vi "COM_Sort_Modes.vi"(7 "Mode":T2, 8 "Error In":errorcluster, 10 "Modes In":T1[](array[typedef]), 11 "Mode Records In":refnum<class "Mode.lvclass">[](array[class])) -> (0 "Error Out":errorcluster, 2 "Modes Out":T1[](array[typedef]), 3 "Mode Records Out":refnum<class "Mode.lvclass">[](array[class]))   [LabVIEW 2017, in "AppPlugins.lvlib" / "EraPlugin.lvclass"]
uses:
  EraPlugin.lvclass
  Mode/Mode.lvclass
  Mode/Mode Content.ctl
  Mode/Mode_Type.ctl
panel:
  in  "Retirement (s)":dbl=30.0 format="%#_13g"
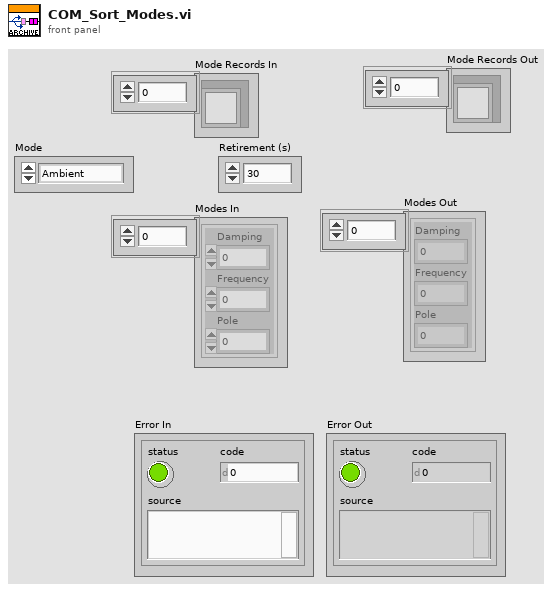
[diagram p1: front panel]
types:
  T1 = typedef "Mode.lvclass/Mode Content.ctl" = cluster{"Damping":dbl, "Frequency":dbl, "Pole":cdb}
  T2 = typedef "Mode.lvclass/Mode_Type.ctl" = enum16{"Ambient", "ERA"}
  T3 = cluster{"avg_f":dbl, "sigma_f":dbl, "avg_d":dbl, "sigma_d":dbl}
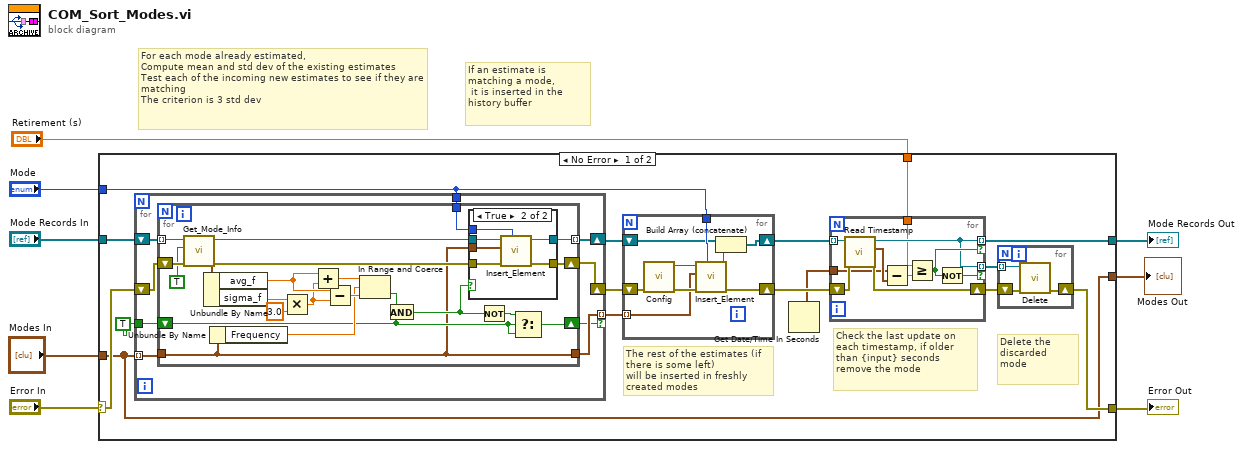
[diagram p0: block diagram]
diagram:
  # "If an estimate is matching a mode,\n it is inserted in the history buffer"
  # "For each mode already estimated,\nCompute mean and std dev of the existing estimates\nTest each of the incoming new estimates to see if they are matching\nThe criterion is 3 std dev"
  n1 = case shown="No Error" "Error In" {
    selector: "Error In" -> [w19 w88]
    tunnel: "Mode Records In" -> [w24 w87]
    tunnel: [w16 w87] -> w7
    tunnel: "Mode" -> [w21 _]
    tunnel: [w12 w88] -> w5
    tunnel: [w9 w86] -> w3
    tunnel: "Retirement (s)" -> [w11 _]
    tunnel: "Modes In" -> [w9 w86]
    frame No Error {
      # "Delete the discarded mode"
      # "Check the last update on each timestamp, if older than {input} seconds remove the mode"
      # "The rest of the estimates (if there is some left) \nwill be inserted in freshly created modes"
      n2 = for {
        shift-right: [w54] -> w22
        shift-left: w19 -> [w51]
        tunnel: w21 -> [w55]
        tunnel: TRUE ("x .and. y?") -> [w53]
        shift-right: [w50] -> w23
        shift-left: w24 -> [w52]
        tunnel: w9 -> [w49] mode=indexing
        tunnel: [w48] -> w10 mode=indexing if=w47
        n3 = for {
          tunnel: w55 -> [w74]
          shift-right: [w73] -> w54
          shift-left: w51 -> [w68]
          shift-right: [w72] -> w47
          shift-left: w53 -> [w62]
          tunnel: w52 -> [w70] mode=indexing
          tunnel: [w65] -> w50 mode=indexing
          tunnel: w49 -> [w56]
          tunnel: [w56] -> w48
          n4 = call "Get_Mode_Info.vi"("Error In"=w68, "Coerce?"=TRUE, "Input"=w70) -> ("Error Out"=w67:errorcluster, "Modes_info"=w66:T3, "Output"=w69:refnum<class "Mode.lvclass">)  [unwired: 5 in, 1 out]
          n5 = Unbundle By Name(w66) -> ("avg_f"=w77:dbl, "sigma_f"=w59:dbl)
          n6 = Unbundle By Name(w56) -> ("Frequency"=w64:dbl)
          n7 = Multiply(x=w59, y=3.0) -> (x*y=w58:dbl)
          n8 = Add(x=w77, y=w58) -> (x+y=w75:dbl)
          n9 = Subtract(x=w77, y=w58) -> (x-y=w76:dbl)
          n10 = In Range and Coerce(upper limit=w75, x=w64, lower limit=w76) -> (In Range?=w63:bool)  [unwired: 1 out]
          n11 = And(x=w63, y=w62) -> (x .and. y?=w61:bool)
          n12 = case shown="True" w61 {
            tunnel: w69 -> [w79 w85]
            tunnel: w74 -> [_ w84]
            tunnel: [w79 w83] -> w65
            tunnel: [w78 w82] -> w73
            tunnel: w67 -> [w78 w81]
            tunnel: w56 -> [_ w80]
            frame False {
            }
            frame True {
              n13 = call "Insert_Element.vi"("Mode"=w84, "Error In"=w81, "New element"=w80, "Input"=w85) -> ("Error Out"=w82:errorcluster, "Output"=w83:refnum<class "Mode.lvclass">)  [unwired: 6 in]
            }
          }
          n14 = Not(x=w61) -> (.not. x?=w71:bool)
          n15 = Select(t=w71, s=w62, f=w62) -> (s? t:f=w72:bool)
        }
      }
      n16 = for {
        tunnel: w10 -> [w38] mode=indexing
        shift-right: [w41] -> w18
        shift-left: w23 -> [w40]
        shift-right: [w43] -> w17
        shift-left: w22 -> [w44]
        tunnel: w21 -> [w42]
        n17 = call "Config.vi"("error in (no error)"=w44) -> ("error out"=w45:errorcluster, "Mode.lvclass"=w46:refnum<class "Mode.lvclass">)  [unwired: 9 in]
        n18 = call "Insert_Element.vi"("Mode"=w42, "Error In"=w45, "New element"=w38, "Input"=w46) -> ("Error Out"=w43:errorcluster, "Output"=w39:refnum<class "Mode.lvclass">)  [unwired: 6 in]
        n19 = Build Array (concatenate)(w40, w39) -> (w41:refnum<class "Mode.lvclass">[])
      }
      n20 = Get Date/Time In Seconds() -> (seconds since 1Jan1904=w15:timestamp)
      n21 = for {
        shift-right: [w36] -> w13
        shift-left: w17 -> [w37]
        tunnel: w18 -> [w35] mode=indexing
        tunnel: [w30] -> w16 mode=indexing if=w31
        tunnel: w15 -> [w33]
        tunnel: [w30] -> w14 mode=indexing if=w29
        tunnel: w11 -> [w28]
        n22 = call-dynamic "Read Timestamp.vi"("error in (no error)"=w37, "Mode in"=w35) -> ("error out"=w36:errorcluster, "last"=w34:timestamp, "Mode out"=w30:refnum<class "Mode.lvclass">)  [unwired: 7 in]
        n23 = Subtract(x=w33, y=w34) -> (x-y=w32:dbl)
        n24 = Greater Or Equal?(x=w28, y=w32) -> (x >= y?=w31:bool)
        n25 = Not(x=w31) -> (.not. x?=w29:bool)
      }
      n26 = for {
        tunnel: w14 -> [w27] mode=indexing
        shift-right: [w25] -> w12
        shift-left: w13 -> [w26]
        n27 = call "Delete.vi"("Error In"=w26, "Mode.lvclass"=w27) -> ("Error Out"=w25:errorcluster)  [unwired: 9 in]
      }
    }
    frame Error {
    }
  }
  "Mode Records Out" <- w7
  "Error Out" <- w5
  "Modes Out" <- w3
